vi "Read Fgen Setting.vi"(8 "error in (no error)":errorcluster, 11 "Fgen configuration":refnum<class "Fgen configuration.lvclass">) -> (0 "error out":errorcluster, 2 "Fgen Setting":T1={"Type"="Arbitrary Waveform", "Output Mode"="Standard Function", "Sample Rate"=10000000.0, "Samples"=1000000.0, "Gain"=1.0, "Trigger"="Start Trigger", "Impedance"="75", "Offset"=0.0} {"Samples" format="%#_6p"; "Sample Rate" format="%#_6p"}, 3 "Fgen configuration out":refnum<class "Fgen configuration.lvclass">)   [LabVIEW 2025, in "Fgen.lvlib" / "Fgen configuration.lvclass"]
uses:
  Fgen configuration.lvclass
  Fgen Setting.ctl
  Fgen configuration.lvclass/Fgen configuration.ctl
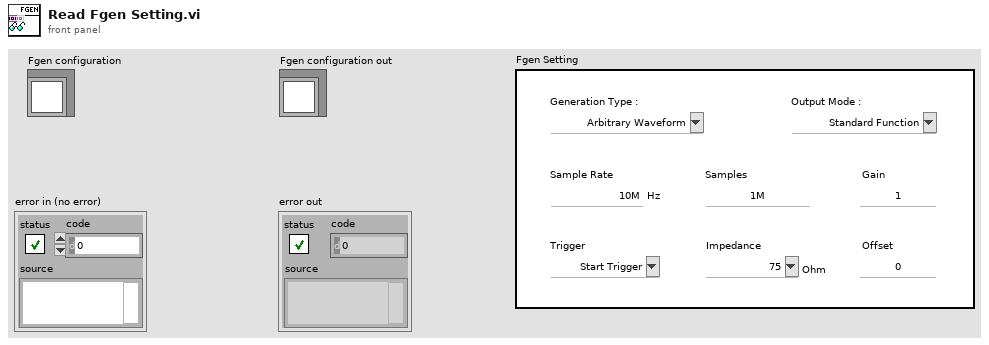
[diagram p1: front panel]
types:
  T1 = typedef "Fgen.lvlib/Fgen configuration.lvclass/Fgen Setting.ctl" = cluster{"Type":string, "Output Mode":string, "Sample Rate":dbl, "Samples":dbl, "Gain":dbl, "Trigger":string, "Impedance":string, "Offset":dbl}
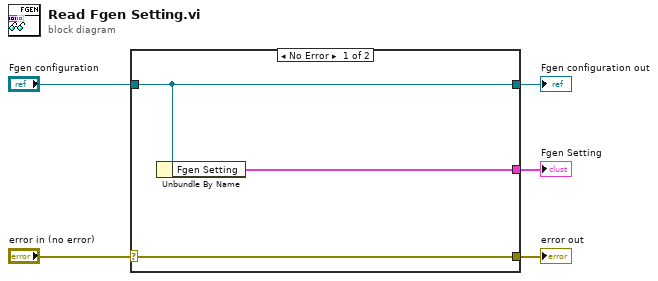
[diagram p0: block diagram]
diagram:
  n1 = case shown="No Error" "error in (no error)" {
    selector: "error in (no error)" -> [w8 w9]
    tunnel: [w8 w9] -> w4
    tunnel: [w7 w10] -> w3
    tunnel: "Fgen configuration" -> [w7 w10]
    tunnel: [w6 _] -> w1
    frame No Error {
      n2 = Unbundle By Name(w7) -> ("Fgen Setting"=w6:T1)
    }
    frame Error {
    }
  }
  "error out" <- w4
  "Fgen configuration out" <- w3
  "Fgen Setting" <- w1
